vi "_PC_DataChrom_XIC2Mass.vi"(7 "Rectangle Allow Index":bool[](array[boolean]), 11 "File path Array":path[](array[path])) -> (1 "Information":string[](array[string]), 3 "DataArray":cluster{"X":dbl[], "Y":dbl[]}[](array[cluster]))   [LabVIEW 2018]
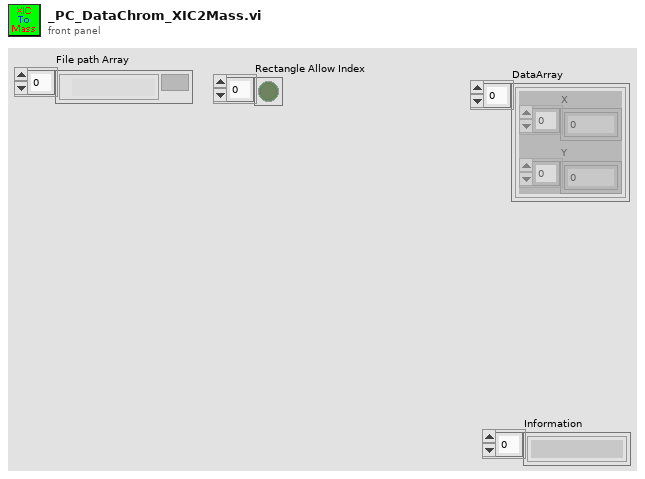
[diagram p1: front panel]
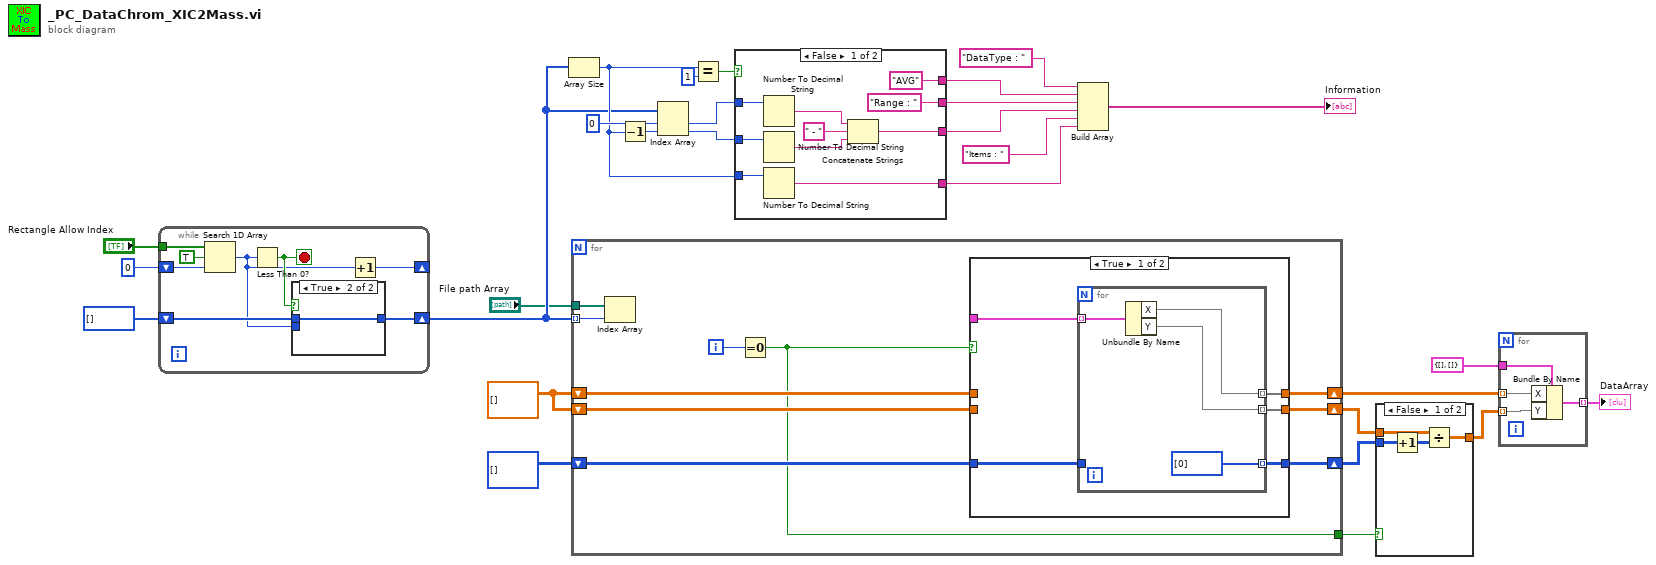
[diagram p0: block diagram]
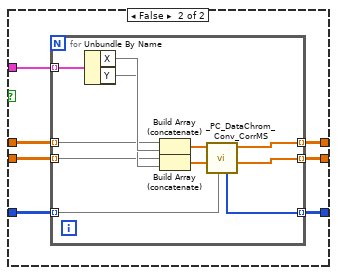
[diagram p2: hidden frame]
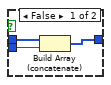
[diagram p3: hidden frame]
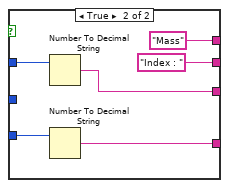
[diagram p4: hidden frame]
diagram:
  w8 = dbl[][] [] ("X")
  n1 = while {
    tunnel: "Rectangle Allow Index" -> [w36]
    shift-right: [w29] -> _
    shift-left: 0 -> [w34]
    shift-right: [w31] -> w2
    shift-left: u32[] [] -> [w33]
    stop <- w32 stop-if-true
    n2 = Search 1D Array(1D array=w36, element=TRUE, start index (0)=w34) -> (index of element=w30:i32)
    n3 = Less Than 0?(x=w30) -> (x < 0?=w32:bool)
    n4 = case shown="True" w32 {
      tunnel: w33 -> [w39 w40]
      tunnel: [w38 w40] -> w31
      tunnel: w30 -> [w37 _]
      frame False {
        n5 = Build Array (concatenate)(w39, w37) -> (w38:u32[])
      }
      frame True {
      }
    }
    n6 = Increment(x=w30) -> (x+1=w29:i32)
  }
  n7 = Array Size(array=w2) -> (size(s)=w10:i32)
  n8 = for {
    tunnel: w2 -> [w50] mode=indexing
    shift-right: [w45] -> w6
    shift-left: w8 -> [w48]
    shift-right: [w44] -> w5
    shift-left: w8 -> [w47]
    shift-right: [w43] -> w4
    shift-left: u16[][] [] ("RepeatTimes_Output") -> [w46]
    tunnel: [w42] -> w3
    tunnel: "File path Array" -> [w41]
    i -> [w49]
    n9 = Index Array(array=w41, index=w50) -> ()  [unwired: 1 out]
    n10 = Equal To 0?(x=w49) -> (x = 0?=w42:bool)
    n11 = case shown="True" w42 {
      tunnel: [w55 w66] -> w45
      tunnel: [w54 w65] -> w44
      tunnel: w48 -> [_ w64]
      tunnel: w47 -> [_ w63]
      tunnel: w46 -> [w53 w62]
      tunnel: [w52 w61] -> w43
      tunnel: _ -> [w51 w60]
      frame True {
        n12 = for {
          tunnel: w51 -> [w59] mode=indexing
          tunnel: [w58] -> w55 mode=indexing
          tunnel: [w57] -> w54 mode=indexing
          tunnel: w53 -> [_]
          tunnel: [u16[] [0]] -> w52 mode=indexing
          n13 = Unbundle By Name(w59) -> ("X"=w58, "Y"=w57)
        }
      }
      frame False {
        n14 = for {
          tunnel: w60 -> [w77] mode=indexing
          tunnel: [w74] -> w66 mode=indexing
          tunnel: [w73] -> w65 mode=indexing
          tunnel: w64 -> [w72] mode=indexing
          tunnel: w63 -> [w71] mode=indexing
          tunnel: w62 -> [w70] mode=indexing
          tunnel: [w69] -> w61 mode=indexing
          n15 = Unbundle By Name(w77) -> ("X"=w76, "Y"=w75)
          n16 = Build Array (concatenate)(w72, w76) -> (w68:dbl[])
          n17 = Build Array (concatenate)(w71, w75) -> (w67:dbl[])
          n18 = call "_PC_DataChrom_Conv_CorrMS.vi"("RepeatTimes_Input"=w70, "Y"=w67, "X"=w68) -> ("Spectrum Y"=w73:dbl[], "Spectrum X"=w74:dbl[], "RepeatTimes_Output"=w69:u16[])  [unwired: 4 in]
        }
      }
    }
  }
  n19 = Decrement(x=w10) -> (x-1=w9:i32)
  n20 = Index Array(array=w2, index #1=0, index #2=w9) -> (element #1=w12:u32, element #2=w11:u32)
  n21 = Equal?(x=w10, y=1) -> (x = y?=w14:bool)
  n22 = case shown="False" w14 {
    tunnel: w11 -> [w84 _]
    tunnel: w12 -> [w85 w91]
    tunnel: w10 -> [w79 w89]
    tunnel: ["AVG" "Mass"] -> w24
    tunnel: ["Range : " "Index : "] -> w23
    tunnel: [w80 w90] -> w22
    tunnel: [w78 w88] -> w20
    frame False {
      n23 = Number To Decimal String(number=w85) -> (decimal integer string=w83:string)  [unwired: 1 in]
      n24 = Number To Decimal String(number=w84) -> (decimal integer string=w81:string)  [unwired: 1 in]
      n25 = Number To Decimal String(number=w79) -> (decimal integer string=w78:string)  [unwired: 1 in]
      n26 = Concatenate Strings(w83, " - ", w81) -> (w80:string)
    }
    frame True {
      n27 = Number To Decimal String(number=w91) -> (decimal integer string=w90:string)  [unwired: 1 in]
      n28 = Number To Decimal String(number=w89) -> (decimal integer string=w88:string)  [unwired: 1 in]
    }
  }
  n29 = Build Array("DataType : ", w24, w23, w22, "Items : ", w20) -> (→"Information":string[])
  n30 = case shown="False" w3 {
    tunnel: w5 -> [w97 w98]
    tunnel: w4 -> [w95 _]
    tunnel: [w96 w98] -> w27
    frame False {
      n31 = Increment(x=w95) -> (x+1=w94:u16[][])
      n32 = Divide(x=w97, y=w94) -> (x/y=w96:dbl[][])
    }
    frame True {
    }
  }
  n33 = for {
    tunnel: w6 -> [w101] mode=indexing
    tunnel: w27 -> [w100] mode=indexing
    tunnel: cluster{"X":dbl[], "Y":dbl[]} {"X"=[], "Y"=[]} ("Data") -> [w102]
    tunnel: [w99] -> w26 mode=indexing
    n34 = Bundle By Name(cluster=w102, "X"=w101, "Y"=w100) -> (w99:cluster{"X":dbl[], "Y":dbl[]})
  }
  "DataArray" <- w26
